vi "GUI - Registration (V1.00).vi"(0 "reference in":refnum<class "Registration.lvclass">, 5 "error in (no error)":errorcluster, 6 "Registration Level IN":T1, 7 "Application Name":string="Regist", 9 "State Queue":string[](array[string])=["SC >>> Initialize", "CTRL >>> KeyGen Mode"]) -> (19 "error out":errorcluster)   [LabVIEW 2022 SP3, in "Registration.lvclass"]
uses:
  Registration.lvclass
  utils/Registration Type.ctl
  W:/projects/archives/23 Charette AI Group/SPWB/API/Generic Utilities_class/Generic Utilities.lvclass
  protected/Registration Info.ctl
  <vilib>/Platform/browser.llb/Open URL in Default Browser (string).vi
  Generic Utilities_class/Generic Utilities.lvclass
  <vilib>/addons/_AddQ/G#Object/G#Object.lvclass
panel:
  in  "Task":enum32{"GUI", "KeyGen", "Settings"}(tab)
  in  "SPWB Home":bool caption="Please click on the button to open the spworkbench Home page and then select the \"Donate\" tab.  Once the donation has been confirmed, you will get an email with the information below, just copy and paste to activate your copy of spworkbench and have access to ALL the features."
  in  "Activation":bool
  in  "Registration Code":string
  in  "Last Name":string
  in  "First Name":string
  in  "Registration Type":T1=enum."Registered - Full Activation"
  out "KeyGen - Customer Code":string
  in  "KeyGen - Last Name":string
  in  "KeyGen - First Name":string
  out "State History":string[](array[string])
  out "State Index":i32=-1
  in  "Exit":bool
  # "For any questions regarding registration, please send an email to: registration@spworkbench.com"
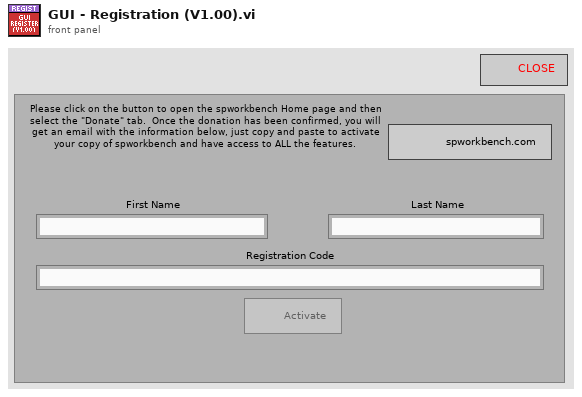
[diagram p1: front panel]
types:
  T1 = typedef "Registration.lvclass/Registration Type.ctl" = enum16{"Unregistered", "Registered - Full Activation", "Not Required- Full Activation"}
  T2 = typedef "Registration.lvclass/Registration Info.ctl" = cluster{"First Name":string, "Last Name":string, "Registration Code":string, "Registration Level":T1}
  T3 = enum8{"Enabled", "Disabled", "Disabled and Grayed Out"}
  T4 = enum32{"Invalid", "Standard", "Closed", "Hidden", "Minimized", "Maximized"}
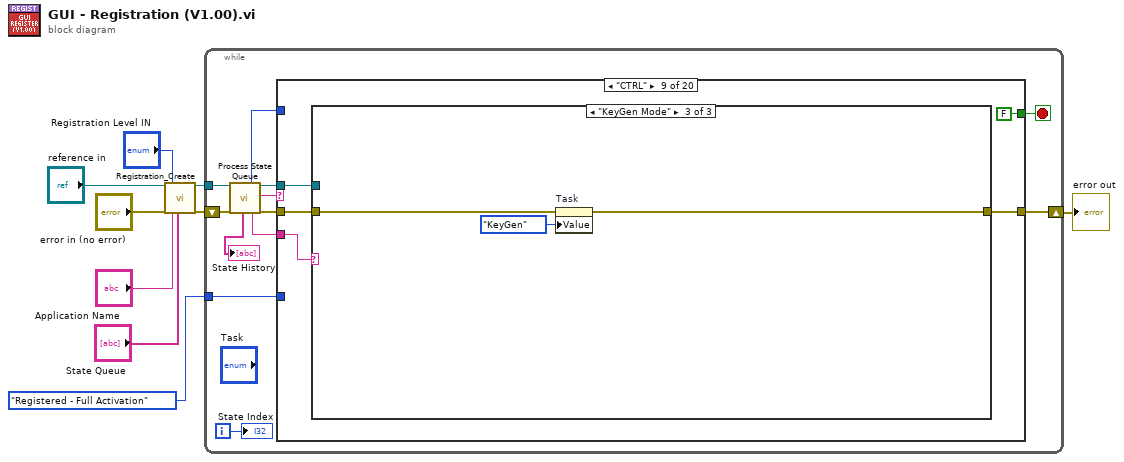
[diagram p0: block diagram]
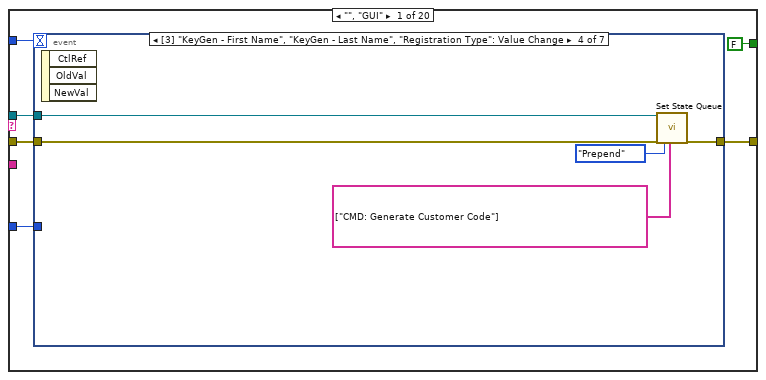
[diagram p2: hidden frame]
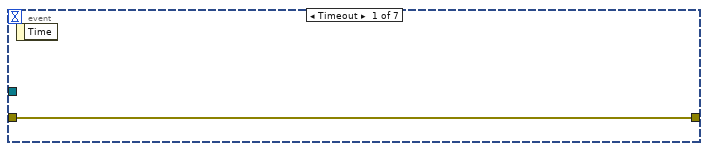
[diagram p3: hidden frame]
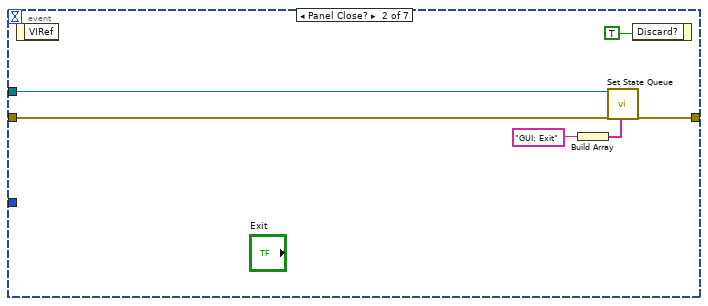
[diagram p4: hidden frame]
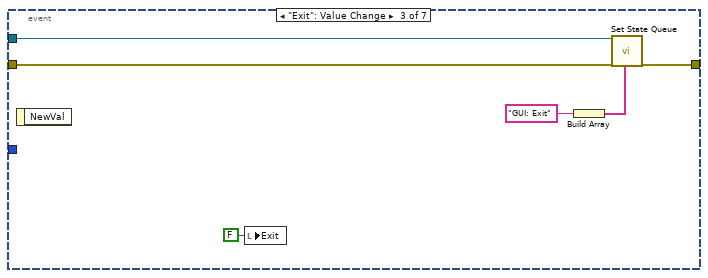
[diagram p5: hidden frame]
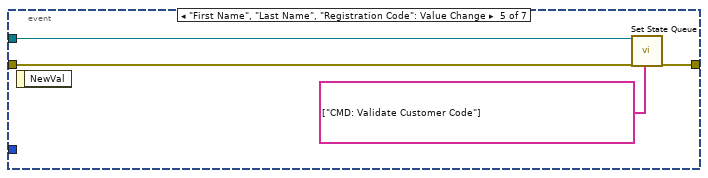
[diagram p6: hidden frame]
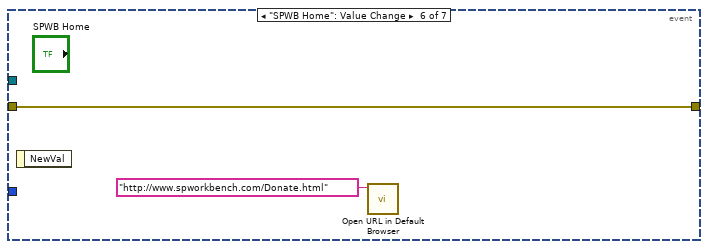
[diagram p7: hidden frame]
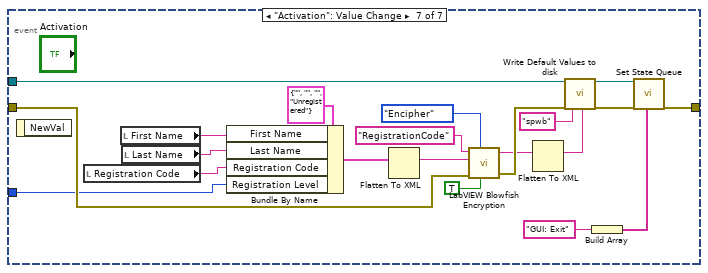
[diagram p8: hidden frame]
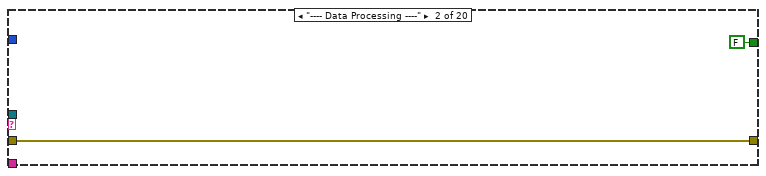
[diagram p9: hidden frame]
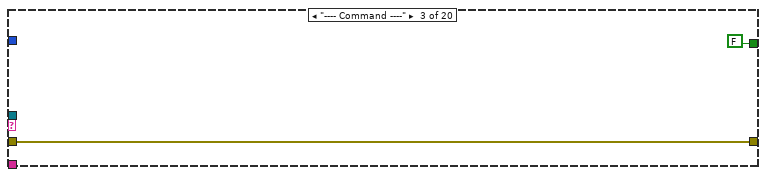
[diagram p10: hidden frame]
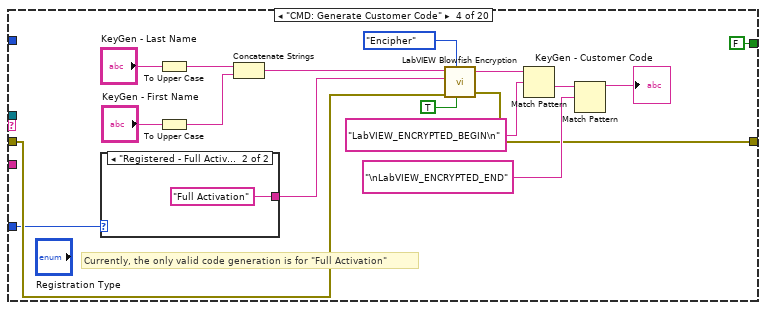
[diagram p11: hidden frame]
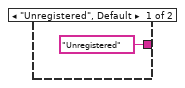
[diagram p12: hidden frame]
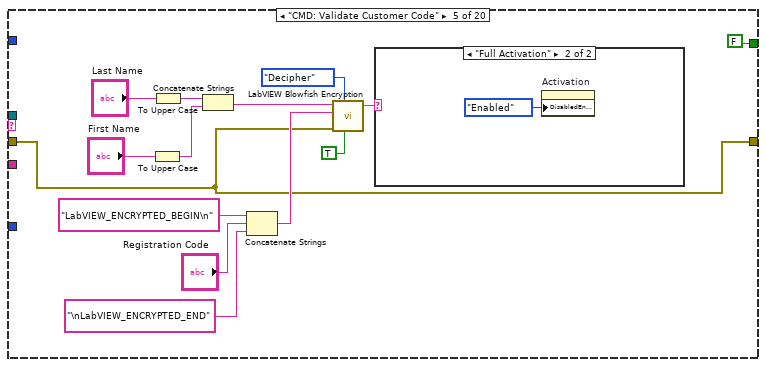
[diagram p13: hidden frame]
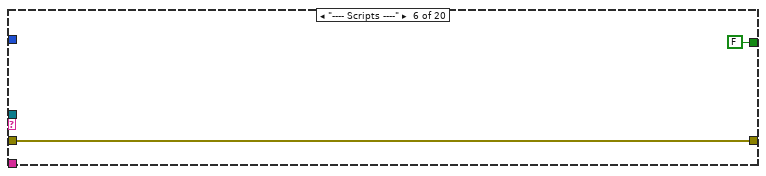
[diagram p15: hidden frame]
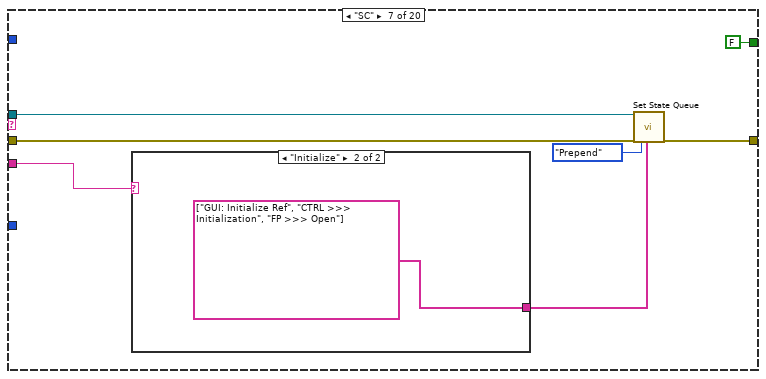
[diagram p16: hidden frame]
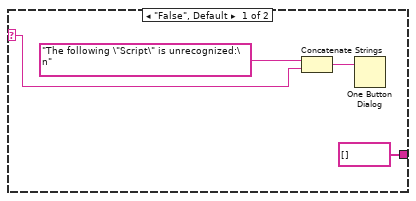
[diagram p17: hidden frame]
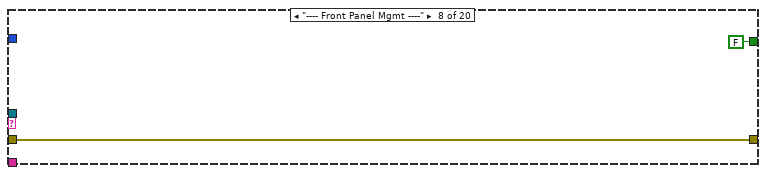
[diagram p18: hidden frame]
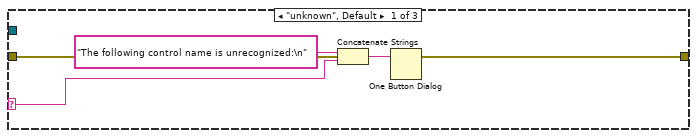
[diagram p19: hidden frame]
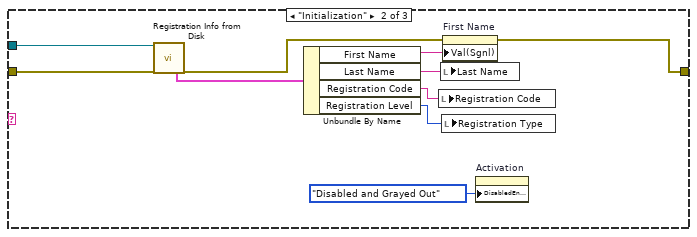
[diagram p20: hidden frame]
diagram:
  n1 = call "Registration_Create.vi"("reference in"="reference in", "error in (no error)"="error in (no error)", "Registration Level"="Registration Level IN", "Application Name"="Application Name", "State Queue"="State Queue") -> ("reference out"=w9:refnum<class "Registration.lvclass">, "error out"=w8:errorcluster)  [unwired: 13 in]
  n2 = while {
    shift-right: [w13] -> w6
    shift-left: w8 -> [w18]
    tunnel: w9 -> [w19]
    tunnel: Registration_Type."Registered - Full Activation" ("Registration Type") -> [w11]
    i -> [w20]
    stop <- w21 stop-if-true
    n3 = call "Process State Queue.vi"("reference in"=w19, "error in (no error)"=w18) -> ("State History"=→"State History":string[], "Timeout"=w17:i32, "State Option"=w12:string, "reference out"=w16:refnum<class "Registration.lvclass">, "Current State"=w15:string, "error out"=w14:errorcluster)  [unwired: 10 in, 2 out]
    n4 = case shown="\"CTRL\"" w15 {
      selector: w15 -> [_ _ _ _ _ _ _ _ _ _ _ _ _ _ _ _ w271 _ _ _]
      tunnel: w16 -> [w25 _ _ _ _ _ w118 _ w129 w152 _ w182 w194 w228 w253 _ _ _ _ w281]
      tunnel: [FALSE FALSE FALSE FALSE FALSE FALSE FALSE FALSE FALSE FALSE FALSE FALSE TRUE FALSE FALSE FALSE FALSE FALSE FALSE TRUE] -> w21
      tunnel: w17 -> [w26 _ _ _ _ _ _ _ _ _ _ _ _ _ _ _ _ _ _ _]
      tunnel: w12 -> [_ _ _ _ _ _ w114 _ w130 w149 _ _ _ w237 _ _ _ _ _ _]
      tunnel: w14 -> [w24 w73 w75 w78 w96 w111 w117 w125 w127 w151 w172 w178 w191 w227 w254 w267 w269 w274 w277 w280]
      tunnel: [w23 w73 w75 w79 w96 w111 w116 w125 w128 w150 w172 w179 w190 w225 w250 w267 w269 errorcluster {"status"=FALSE, "code"=0, "source"=""} ("error out") w277 w279] -> w13
      tunnel: w11 -> [w22 _ _ w77 _ _ _ _ _ _ _ _ _ _ _ _ _ _ _ _]
      frame "", "GUI" {
        n5 = event shown="[3] \"KeyGen - First Name\", \"KeyGen - Last Name\", \"Registration Type\": Value Change" {
          selector: _ -> [_ _ _ _ _ _ _]
          dyn-events: _ -> [_ _ _ _ _ _ _]
          timeout: w26 -> [_ _ _ _ _ _ _]
          tunnel: w25 -> [_ w32 w38 w44 w48 _ w67]
          tunnel: w24 -> [w28 w31 w36 w43 w47 w51 w62]
          tunnel: [w28 w30 w37 w45 w49 w51 w52] -> w23
          tunnel: w22 -> [_ _ _ _ _ _ w57]
          event Timeout {
            n6 = event-data() -> ()  [unwired: 1 in, 1 out]
          }
          event Panel Close? {
            n7 = event-data() -> ()  [unwired: 1 in, 1 out]
            n8 = Build Array("GUI: Exit") -> (w29:string[])
            n9 = call "Set State Queue.vi"("reference in"=w32, "error in (no error)"=w31, "State Queue"=w29) -> ("error out"=w30:errorcluster)  [unwired: 15 in, 1 out]
            n10 = event-data("Discard?"=TRUE) -> ()  [unwired: 1 in, 1 out]
          }
          event "Exit": Value Change {
            n11 = event-data() -> ()  [unwired: 1 in, 1 out]
            n12 = local write "Exit"(FALSE ("Exit")) -> ()
            n13 = Build Array("GUI: Exit") -> (w35:string[])
            n14 = call "Set State Queue.vi"("reference in"=w38, "error in (no error)"=w36, "State Queue"=w35) -> ("error out"=w37:errorcluster)  [unwired: 15 in, 1 out]
          }
          event "KeyGen - First Name", "KeyGen - Last Name": Value Change {
            n15 = event-data() -> ()  [unwired: 1 in, 3 out]
            n16 = call "Set State Queue.vi"("reference in"=w44, "error in (no error)"=w43, "State Queue Options"=enum16{"Replace", "Append", "Prepend"}."Prepend", "State Queue"=string[] ["CMD: Generate Customer Code"] ("State Queue OUT")) -> ("error out"=w45:errorcluster)  [unwired: 14 in, 1 out]
          }
          event "First Name", "Last Name", "Registration Code": Value Change {
            n17 = event-data() -> ()  [unwired: 1 in, 1 out]
            n18 = call "Set State Queue.vi"("reference in"=w48, "error in (no error)"=w47, "State Queue"=string[] ["CMD: Validate Customer Code"] ("State Queue OUT")) -> ("error out"=w49:errorcluster)  [unwired: 15 in, 1 out]
          }
          event "SPWB Home": Value Change {
            n19 = event-data() -> ()  [unwired: 1 in, 1 out]
            n20 = call-poly <vilib>:"Open URL in Default Browser.vi"("URL"="http://www.spworkbench.com/Donate.html") -> ()  [unwired: 5 in, 2 out]
          }
          event "Activation": Value Change {
            n21 = event-data() -> ()  [unwired: 1 in, 1 out]
            n22 = local read "Registration Code"() -> (w70:string)
            n23 = local read "First Name"() -> (w72:string)
            n24 = local read "Last Name"() -> (w71:string)
            n25 = Bundle By Name(cluster=T2 {"First Name"="", "Last Name"="", "Registration Code"="", "Registration Level"=enum."Unregistered"} ("Registration Info"), "First Name"=w72, "Last Name"=w71, "Registration Code"=w70, "Registration Level"=w57) -> (w65:T2)
            n26 = Flatten To XML(6:w65) -> (2:w64:string)
            n27 = call "LabVIEW Blowfish Encryption.vi"("Password"="RegistrationCode", "Enc/Dec"=enum16{"Encipher", "Decipher"}."Encipher", "Input Text"=w64, "Output As ASCII\nfor email Transmission"=TRUE ("Output As ASCII\nfor email Transmission"), "error in (no error)"=w62) -> ("Output text"=w59:string, "error out"=w61:errorcluster)  [unwired: 1 in, 1 out]
            n28 = Flatten To XML(6:w59) -> (2:w58:string)
            n29 = call-dynamic "Write Default Values to disk.vi"("reference in"=w67, "error in (no error)"=w61, "Control Label"="spwb" ("Filename"), "Value (XML String)"=w58) -> ("reference out"=w53:refnum<class "Registration.lvclass">, "error out"=w54:errorcluster)  [unwired: 14 in]
            n30 = Build Array("GUI: Exit") -> (w55:string[])
            n31 = call "Set State Queue.vi"("reference in"=w53, "error in (no error)"=w54, "State Queue"=w55) -> ("error out"=w52:errorcluster)  [unwired: 15 in, 1 out]
          }
        }
      }
      frame "---- Data Processing ----" {
      }
      frame "---- Command ----" {
      }
      frame "CMD: Generate Customer Code" {
        # "Currently, the only valid code generation is for \"Full Activation\""
        n32 = case shown="\"Registered - Full Activation\"" w77 {
          tunnel: ["Unregistered" ("Input Text") "Full Activation" ("Input Text")] -> w80
          frame "Unregistered", Default {
          }
          frame "Registered - Full Activation" {
          }
        }
        n33 = To Upper Case(1:"KeyGen - Last Name") -> (0:w90:string)
        n34 = To Upper Case(1:"KeyGen - First Name") -> (0:w91:string)
        n35 = Concatenate Strings(w90, w91) -> (w82:string)
        n36 = call "LabVIEW Blowfish Encryption.vi"("Password"=w82, "Enc/Dec"=enum16{"Encipher", "Decipher"}."Encipher", "Input Text"=w80, "Output As ASCII\nfor email Transmission"=TRUE ("Output As ASCII\nfor email Transmission"), "error in (no error)"=w78) -> ("Output text"=w84:string, "error out"=w79:errorcluster)  [unwired: 1 in, 1 out]
        n37 = Match Pattern(string=w84, regular expression="LabVIEW_ENCRYPTED_BEGIN\n" ("Input Text")) -> (after substring=w86:string)  [unwired: 1 in, 3 out]
        n38 = Match Pattern(string=w86, regular expression="\nLabVIEW_ENCRYPTED_END" ("Input Text")) -> (before substring=→"KeyGen - Customer Code":string)  [unwired: 1 in, 3 out]
      }
      frame "CMD: Validate Customer Code" {
        n39 = To Upper Case(1:"First Name") -> (0:w108:string)
        n40 = To Upper Case(1:"Last Name") -> (0:w107:string)
        n41 = Concatenate Strings(w107, w108) -> (w104:string)
        n42 = Concatenate Strings("LabVIEW_ENCRYPTED_BEGIN\n" ("Input Text"), "Registration Code", "\nLabVIEW_ENCRYPTED_END" ("Input Text")) -> (w100:string)
        n43 = call "LabVIEW Blowfish Encryption.vi"("Password"=w104, "Enc/Dec"=enum16{"Encipher", "Decipher"}."Decipher", "Input Text"=w100, "Output As ASCII\nfor email Transmission"=TRUE ("Output As ASCII\nfor email Transmission"), "error in (no error)"=w96) -> ("Output text"=w97:string)  [unwired: 1 in, 2 out]
        n44 = case shown="\"Full Activation\"" w97 {
          frame "Unregistered", Default {
          }
          frame "Full Activation" {
            n45 = property on="Activation" class="Bool"("DisabledEnum"=T3."Enabled" ("Disabled")) -> ()  [unwired: 2 in, 2 out]
          }
        }
      }
      frame "---- Scripts ----" {
      }
      frame "SC" {
        n46 = case shown="\"Initialize\"" w114 {
          selector: w114 -> [w121 _]
          tunnel: [string[] [] ("State Queue OUT") string[] ["GUI: Initialize Ref", "CTRL >>> Initialization", "FP >>> Open"] ("State Queue OUT")] -> w115
          frame "False", Default {
            n47 = Concatenate Strings("The following \"Script\" is unrecognized:\n", w121) -> (w122:string)
            n48 = One Button Dialog(message=w122) -> ()  [unwired: 1 in, 1 out]
          }
          frame "Initialize" {
          }
        }
        n49 = call "Set State Queue.vi"("reference in"=w118, "error in (no error)"=w117, "State Queue Options"=enum16{"Replace", "Append", "Prepend"}."Prepend", "State Queue"=w115) -> ("error out"=w116:errorcluster)  [unwired: 14 in, 1 out]
      }
      frame "---- Front Panel Mgmt ----" {
      }
      frame "CTRL" {
        n50 = case shown="\"KeyGen Mode\"" w130 {
          selector: w130 -> [w134 _ _]
          tunnel: w129 -> [_ w145 _]
          tunnel: [w132 w138 w147] -> w128
          tunnel: w127 -> [w132 w144 w148]
          frame "unknown", Default {
            n51 = Concatenate Strings("The following control name is unrecognized:\n", w134) -> (w133:string)
            n52 = One Button Dialog(message=w133) -> ()  [unwired: 1 in, 1 out]
          }
          frame "Initialization" {
            n53 = call "Registration Info from Disk.vi"("reference in"=w145, "error in (no error)"=w144) -> ("Registration Info"=w136:T2, "error out"=w139:errorcluster)  [unwired: 15 in, 1 out]
            n54 = Unbundle By Name(w136) -> ("First Name"=w140:string, "Last Name"=w143:string, "Registration Code"=w141:string, "Registration Level"=w142:T1)
            n55 = local write "Registration Code"(w141) -> ()
            n56 = local write "Last Name"(w143) -> ()
            n57 = local write "Registration Type"(w142) -> ()
            n58 = property on="First Name" class="Str"(error in=w139, "Val(Sgnl)"=w140) -> (error out=w138:errorcluster)  [unwired: 1 in, 1 out]
            n59 = property on="Activation" class="Bool"("DisabledEnum"=T3."Disabled and Grayed Out" ("Disabled")) -> ()  [unwired: 2 in, 2 out]
          }
          frame "KeyGen Mode" {
            n60 = property on="Task" class="TabCtl (strict)"(error in=w148, "Value"=enum32{"GUI", "KeyGen", "Settings"}."KeyGen" ("Task")) -> (error out=w147:errorcluster)  [unwired: 1 in, 1 out]
          }
        }
      }
      frame "FP" {
        n61 = case shown="\"Open\"" w149 {
          selector: w149 -> [w154 _]
          tunnel: w152 -> [_ w162]
          tunnel: w151 -> [w155 w161]
          tunnel: [w155 w158] -> w150
          frame "unknown", Default {
            n62 = Concatenate Strings("The following FP Command name is unrecognized:\n", w154) -> (w156:string)
            n63 = One Button Dialog(message=w156) -> ()  [unwired: 1 in, 1 out]
          }
          frame "Open" {
            n64 = call-dynamic "Get VI Ref.vi"("reference in"=w162, "error in (no error)"=w161) -> ("GUI VI Ref"=w159:refnum<vi>, "error out"=w160:errorcluster)  [unwired: 14 in, 2 out]
            n65 = property class="VI"(reference=w159, error in=w160) -> (reference out=w164:refnum<vi>, error out=w165:errorcluster, "Front Panel.Open"=w163:bool)
            n66 = case shown="True" w163 {
              tunnel: [w168 w171] -> w158
              tunnel: w165 -> [w167 w171]
              tunnel: w164 -> [w166 _]
              frame False {
                n67 = invoke class="VI" method="FP.Open"(reference=w166, error in=w167, "Activate"=TRUE, "State"=T4."Standard") -> (error out=w168:errorcluster)  [unwired: 1 in, 4 out]
              }
              frame True {
              }
            }
          }
        }
      }
      frame "---- GUI Functions ----" {
      }
      frame "GUI: Initialize Ref" {
        n68 = control-ref of="GUI Reference"() -> (w177:refnum<vi>)
        n69 = call "Set VI Ref.vi"("reference in"=w182, "error in (no error)"=w178, "ReInit All to Default?"=TRUE, "GUI VI Ref"=w177) -> ("reference out"=w181:refnum<class "Registration.lvclass">, "error out"=w176:errorcluster)  [unwired: 14 in]
        n70 = call "Set Close Panel (Yes or No).vi"("reference in"=w181, "error in (no error)"=w176) -> ("reference out"=w180:refnum<class "Registration.lvclass">, "error out"=w175:errorcluster)  [unwired: 16 in]
        n71 = call "Set Message Window Ref.vi"("reference in"=w180, "error in (no error)"=w175) -> ("error out"=w179:errorcluster)  [unwired: 16 in, 1 out]
      }
      frame "GUI: Exit" {
        n72 = call-dynamic "Get Message Window Ref.vi"("reference in"=w194, "error in (no error)"=w191) -> ("reference out"=w193:refnum<class "Registration.lvclass">, "Msg Win Ref"=w189:refnum<vi>, "error out"=w192:errorcluster)  [unwired: 15 in]
        n73 = call-dynamic "Get VI Ref.vi"("reference in"=w193, "error in (no error)"=w192) -> ("reference out"=w198:refnum<class "Registration.lvclass">, "GUI VI Ref"=w196:refnum<vi>, "error out"=w197:errorcluster)  [unwired: 14 in, 1 out]
        n74 = call-dynamic "Get Close Panel (Yes or No).vi"("reference in"=w198, "error in (no error)"=w197) -> ("Close Panel?"=w199:bool, "reference out"=w188:refnum<class "Registration.lvclass">, "error out"=w187:errorcluster)  [unwired: 15 in]
        n75 = call "Get - Object Origin.vi"("reference in"=w188, "error in (no error)"=w187) -> ("Object Origin"=w184:enum16{"New/Created", "Existing"}, "reference out"=w186:refnum<class "Registration.lvclass">, "error out"=w185:errorcluster)  [unwired: 15 in]
        n76 = case shown="\"Existing\"" w184 {
          tunnel: [w207 w208] -> w195
          tunnel: w186 -> [w205 _]
          tunnel: w185 -> [w204 w208]
          frame "New/Created", Default {
            n77 = call-dynamic "Destroy.vi"("reference in"=w205, "error in (no error)"=w204) -> ("error out"=w206:errorcluster)  [unwired: 16 in, 1 out]
            n78 = call <vilib>:"GarbageCollector.vi"("error in (no error)"=w206) -> ("error out"=w207:errorcluster)  [unwired: 16 in, 2 out]
          }
          frame "Existing" {
          }
        }
        n79 = Close Reference(reference=w189, error in (no error)=w195) -> (error out=w202:errorcluster)
        n80 = case shown="True" w199 {
          tunnel: w202 -> [w210 w214]
          tunnel: [w210 w213] -> w200
          tunnel: [w209 w212] -> w201
          tunnel: w196 -> [w209 w211]
          frame False {
          }
          frame True {
            n81 = property class="VI"(reference=w211, error in=w214) -> (reference out=w216:refnum<vi>, error out=w215:errorcluster, "Front Panel.Open"=w217:bool)
            n82 = case shown="False" w217 {
              tunnel: [w219 w223] -> w213
              tunnel: w215 -> [w219 w222]
              tunnel: w216 -> [w218 w221]
              tunnel: [w218 w220] -> w212
              frame False {
              }
              frame True {
                n83 = invoke class="VI" method="FP.Close"(reference=w221, error in=w222) -> (reference out=w220:refnum<vi>, error out=w223:errorcluster)  [unwired: 1 in, 1 out]
              }
            }
          }
        }
        n84 = Close Reference(reference=w201, error in (no error)=w200) -> (error out=w190:errorcluster)
      }
      frame "SEND MSG" {
        n85 = call-dynamic "Get Message Window Ref.vi"("reference in"=w228, "error in (no error)"=w227) -> ("Msg Win Ref"=w224:refnum<vi>, "error out"=w226:errorcluster)  [unwired: 15 in, 1 out]
        n86 = property class="VI"(reference=w224, error in=w226) -> (reference out=w230:refnum<vi>, error out=w229:errorcluster, "Front Panel.Open"=w231:bool)
        n87 = case shown="False" w231 {
          tunnel: [w245 w249] -> w233
          tunnel: w229 -> [w240 w249]
          tunnel: w230 -> [w242 w248]
          tunnel: [w244 w248] -> w232
          frame False {
            w243 = FALSE ("Wait Until Done")
            n88 = invoke class="VI" method="Run VI"(reference=w242, error in=w240, "Wait until done"=w243, "Auto Dispose Ref"=w243) -> (reference out=w241:refnum<vi>, error out=w239:errorcluster)  [unwired: 1 in, 3 out]
            n89 = invoke class="VI" method="FP.Open"(reference=w241, error in=w239, "Activate"=TRUE, "State"=T4."Standard") -> (reference out=w244:refnum<vi>, error out=w245:errorcluster)  [unwired: 1 in, 3 out]
          }
          frame True {
          }
        }
        n90 = Concatenate Strings("\r\n", w237) -> (w236:string)
        n91 = invoke class="VI" method="Ctrl Val.Set"(reference=w232, error in=w233, "Control Name"="Message", "Value"=w236) -> (error out=w225:errorcluster)  [unwired: 1 in, 4 out]
      }
      frame "CLOSE MSG" {
        n92 = call-dynamic "Get Message Window Ref.vi"("reference in"=w253, "error in (no error)"=w254) -> ("Msg Win Ref"=w251:refnum<vi>, "error out"=w252:errorcluster)  [unwired: 15 in, 1 out]
        n93 = property class="VI"(reference=w251, error in=w252) -> (reference out=w258:refnum<vi>, error out=w259:errorcluster, "Front Panel.Open"=w257:bool)
        n94 = case shown="True" w257 {
          tunnel: [w262 w266] -> w256
          tunnel: w259 -> [w262 w265]
          tunnel: w258 -> [w261 w264]
          tunnel: [w261 w263] -> w255
          frame False {
          }
          frame True {
            n95 = invoke class="VI" method="FP.Close"(reference=w264, error in=w265) -> (reference out=w263:refnum<vi>, error out=w266:errorcluster)  [unwired: 1 in, 1 out]
          }
        }
        n96 = invoke class="VI" method="Abort VI"(reference=w255, error in=w256) -> (error out=w250:errorcluster)  [unwired: 1 in, 2 out]
      }
      frame "---- Miscelleneous ----" {
      }
      frame "unknown", Default {
        n97 = Concatenate Strings("The following state is unrecognized?\n", w271) -> (w270:string)
        n98 = One Button Dialog(message=w270) -> ()  [unwired: 1 in, 1 out]
      }
      frame "Error" {
        n99 = call <vilib>:"General Error Handler.vi"("error in (no error)"=w274) -> ()  [unwired: 10 in, 5 out]
      }
      frame "Next" {
        # "This is an empty case used so the queue does NOT stop if there is an empty string between two valid states!"
      }
      frame "Quit" {
        # "WARNING!, If the state machine crash, then it will also \"Quit\"??"
        # "This is the case used to simply exit when this GUI is used as a SubVI!"
        n100 = call-dynamic "Destroy.vi"("reference in"=w281, "error in (no error)"=w280) -> ("error out"=w279:errorcluster)  [unwired: 16 in, 1 out]
      }
    }
    "State Index" <- w20
  }
  "error out" <- w6
